vi "meta_closeMetaFile.vi"(8 "error in (no error)":errorcluster, 11 "meta file in":T1) -> (0 "error out":errorcluster, 3 "path":path)   [LabVIEW 2017, in "NI_ExcelFile.lvlib"]
uses:
  <vilib>/express/express shared/NI_ExcelFile/NI_ExcelFile.lvlib
  <vilib>/express/express shared/NI_ExcelFile/Ctrls/meta_file.ctl
  <vilib>/express/express shared/NI_ExcelFile/Ctrls/meta_Block.ctl
  <vilib>/express/express shared/NI_ExcelFile/Ctrls/meta_BlockType.ctl
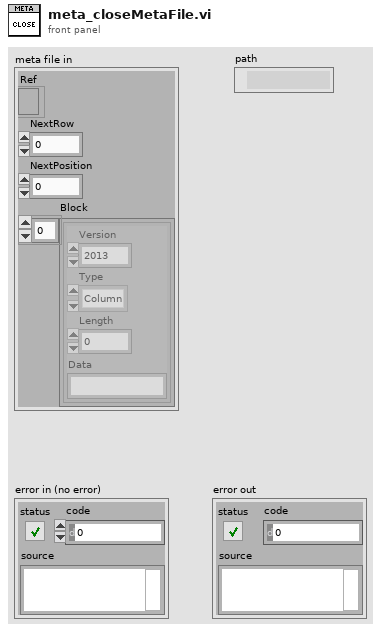
[diagram p1: front panel]
types:
  T1 = typedef "NI_ExcelFile.lvlib/meta_file.ctl" = cluster{"Ref":refnum<file>, "NextRow":i32, "NextPosition":i64, "Block":T2[]}
  T2 = typedef "NI_ExcelFile.lvlib/meta_Block.ctl" = cluster{"Version":u16, "Type":T3, "Length":i32, "Data":string}
  T3 = typedef "NI_ExcelFile.lvlib/meta_BlockType.ctl" = enum16{"NITag", "File", "Column"}
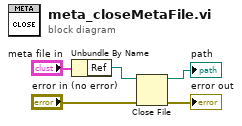
[diagram p0: block diagram]
diagram:
  n1 = Unbundle By Name("meta file in") -> ("Ref"=w1:refnum<file>)
  n2 = Close File(refnum=w1, error in="error in (no error)") -> (path=→"path":path, error out=→"error out":errorcluster)
